vi "in_ensure monotonic.vi"(8 "X is monotonic":bool, 10 "Y":dbl[](array[numeric]), 11 "X":dbl[](array[numeric])) -> (2 "Y out":dbl[](array[numeric]), 3 "X out":dbl[](array[numeric]))   [LabVIEW 2020, in "NI_Gmath.lvlib"]
uses:
  <vilib>/gmath/NI_Gmath.lvlib
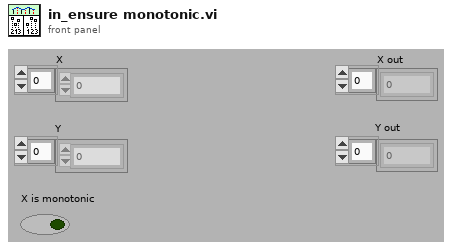
[diagram p1: front panel]
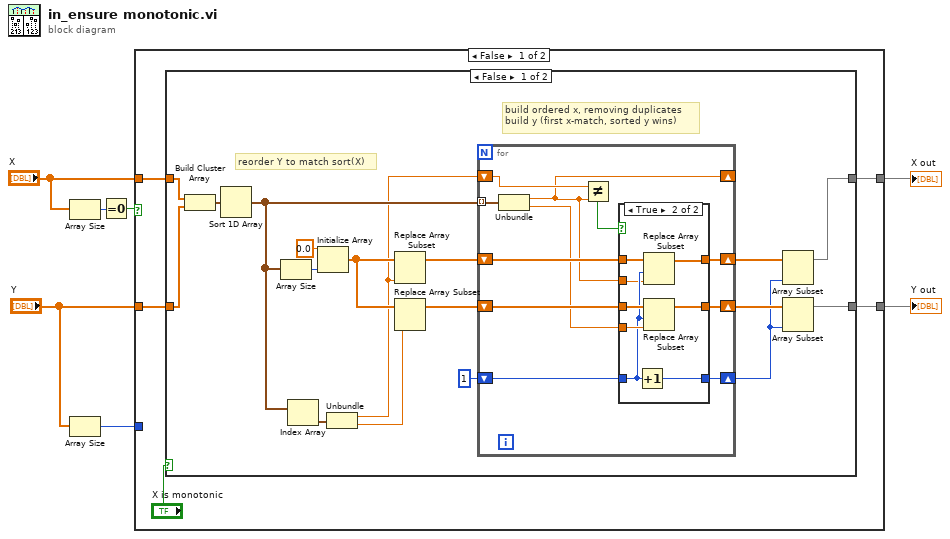
[diagram p0: block diagram]
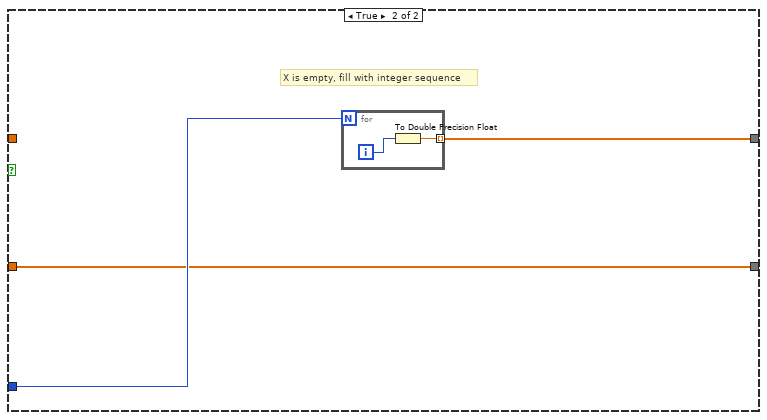
[diagram p4: hidden frame]
diagram:
  n1 = Array Size(array="X") -> (size(s)=w7:i32)
  n2 = Array Size(array="Y") -> (size(s)=w6:i32)
  n3 = Equal To 0?(x=w7) -> (x = 0?=w5:bool)
  n4 = case shown="False" w5 {
    tunnel: w6 -> [_ w57]
    tunnel: [w10 w55] -> w2
    tunnel: "X" -> [w12 _]
    tunnel: [w9 w56] -> w3
    tunnel: "Y" -> [w11 w55]
    frame False {
      n5 = case shown="False" "X is monotonic" {
        tunnel: w12 -> [w29 w53]
        tunnel: w11 -> [w28 w54]
        tunnel: [w14 w54] -> w10
        tunnel: [w15 w53] -> w9
        frame False {
          # "build ordered x, removing duplicates\nbuild y (first x-match, sorted y wins)"
          # "reorder Y to match sort(X)"
          n6 = Build Cluster Array(w29, w28) -> (w30:cluster{"Numeric":dbl, "Numeric":dbl}[])
          n7 = Sort 1D Array(array=w30) -> (sorted array=w22:cluster{"Numeric":dbl, "Numeric":dbl}[])
          n8 = Array Size(array=w22) -> (size(s)=w26:i32)
          n9 = Index Array(array=w22) -> (element=w27:cluster{"Numeric":dbl, "Numeric":dbl})  [unwired: 1 in]
          n10 = Initialize Array(0.0 ("Numeric"), w26) -> (w23:dbl[])
          n11 = Unbundle(w27) -> ("Numeric"=w21:dbl, "Numeric"=w24:dbl)
          n12 = Replace Array Subset(array=w23, new element=w21) -> (w20:dbl[])  [unwired: 1 in]
          n13 = Replace Array Subset(array=w23, new element=w24) -> (w19:dbl[])  [unwired: 1 in]
          n14 = for {
            tunnel: w22 -> [w41] mode=indexing
            shift-right: [w36] -> w18
            shift-left: w20 -> [w40]
            shift-right: [w35] -> w17
            shift-left: w19 -> [w39]
            shift-right: [w31] -> _
            shift-left: w21 -> [w34]
            shift-right: [w32] -> w13
            shift-left: 1 -> [w33]
            n15 = Unbundle(w41) -> ("Numeric"=w31:dbl, "Numeric"=w38:dbl)
            n16 = Not Equal?(x=w34, y=w31) -> (x != y?=w37:bool)
            n17 = case shown="True" w37 {
              tunnel: w40 -> [w44 w52]
              tunnel: w39 -> [w43 w51]
              tunnel: w31 -> [_ w45]
              tunnel: w38 -> [_ w47]
              tunnel: [w44 w50] -> w36
              tunnel: [w43 w49] -> w35
              tunnel: w33 -> [w42 w46]
              tunnel: [w42 w48] -> w32
              frame False {
              }
              frame True {
                n18 = Increment(x=w46) -> (x+1=w48:i32)
                n19 = Replace Array Subset(array=w52, new element=w45, index=w46) -> (w50:dbl[])
                n20 = Replace Array Subset(array=w51, new element=w47, index=w46) -> (w49:dbl[])
              }
            }
          }
          n21 = Array Subset(array=w18, length=w13) -> (w15:dbl[])  [unwired: 1 in]
          n22 = Array Subset(array=w17, length=w13) -> (w14:dbl[])  [unwired: 1 in]
        }
        frame True {
        }
      }
    }
    frame True {
      # "X is empty, fill with integer sequence"
      n23 = for {
        N: w57 -> [_]
        tunnel: [w58] -> w56 mode=indexing
        i -> [w59]
        n24 = To Double Precision Float(number=w59) -> (double precision float=w58:dbl)
      }
    }
  }
  "X out" <- w3
  "Y out" <- w2
